vi "Winch Globals.vi"() -> ()   [LabVIEW 2016]
panel:
  in  "Winch In Angle":dbl
  in  "Winch Out Angle":dbl
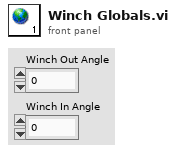
[diagram p1: front panel]
diagram:
